vi "set default pixel clock.vi"(8 "error in (no error)":errorcluster, 11 "Thorcam in":refnum<class "Thorcam.lvclass">) -> (0 "error out":errorcluster, 1 "pixel clock":dbl[unit], 3 "Thorcam out":refnum<class "Thorcam.lvclass">)   [LabVIEW 2012, in "Thorcam.lvclass"]
uses:
  Thorcam.lvclass
  Thorcam.lvclass/Thorcam.ctl
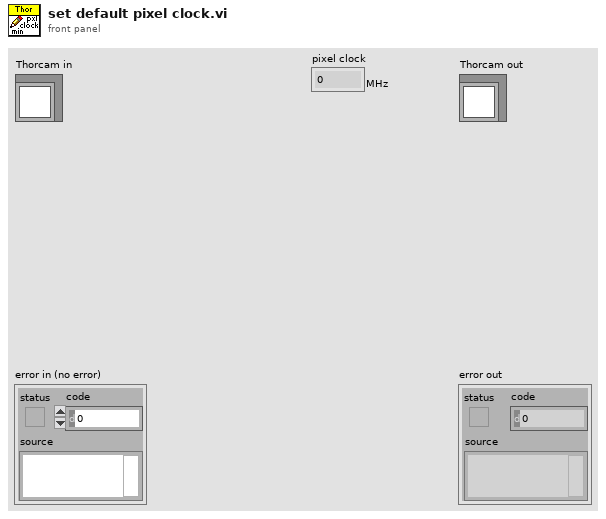
[diagram p1: front panel]
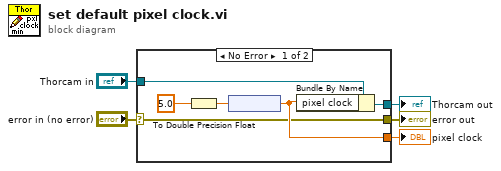
[diagram p0: block diagram]
diagram:
  n1 = case shown="No Error" "error in (no error)" {
    selector: "error in (no error)" -> [w7 w13]
    tunnel: [w7 w13] -> w4
    tunnel: [w10 w12] -> w2
    tunnel: "Thorcam in" -> [w11 w12]
    tunnel: [w9 _] -> w1
    frame No Error {
      n2 = To Double Precision Float(number=5.0) -> (double precision float=w8:dbl)
      n3 = node(w8) -> (w9:dbl[unit])
      n4 = Bundle By Name(cluster=w11, "pixel clock"=w9) -> (w10:refnum<class "Thorcam.lvclass">)
    }
    frame Error {
    }
  }
  "error out" <- w4
  "Thorcam out" <- w2
  "pixel clock" <- w1
